vi "oa_Get Angular Speed (N Tach).vi"(7 "reset? (True)":bool=TRUE, 8 "error in (no error)":errorcluster, 9 "durations":dbl[](array[numeric]), 10 "pulse/revolution (1)":i32[](array[numeric]), 11 "pulse position [s]":cluster{dbl[]}[](array[cluster]) {"?" format="%.2f"}) -> (0 "error out":errorcluster, 1 "No Tach? (False)":bool[](array[boolean]), 2 "speed position info":T2[](array[typedef]), 3 "speed profile":T1[](array[typedef]) {"speed [RPM]" format="%.2f"; "time [s]" format="%.2f"})   [LabVIEW 2017, in "SoundVib_TachProcess.lvlib"]
uses:
  <vilib>/addons/Sound and Vibration/Order Analysis/Tach Process/SoundVib_TachProcess.lvlib
  <vilib>/addons/Sound and Vibration/Order Analysis/Misc/OAT Position Info.ctl
  <vilib>/addons/Sound and Vibration/Order Analysis/Tach Process/SubVIs/speed profile.ctl
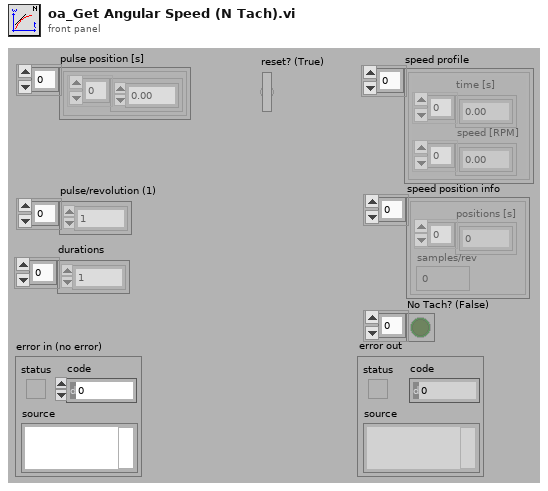
[diagram p1: front panel]
types:
  T1 = typedef "SoundVib_TachProcess.lvlib/speed profile.ctl" = cluster{"time [s]":dbl[], "speed [RPM]":dbl[]}
  T2 = typedef "OAT Position Info.ctl" = cluster{"positions [s]":dbl[], "samples/rev":dbl}
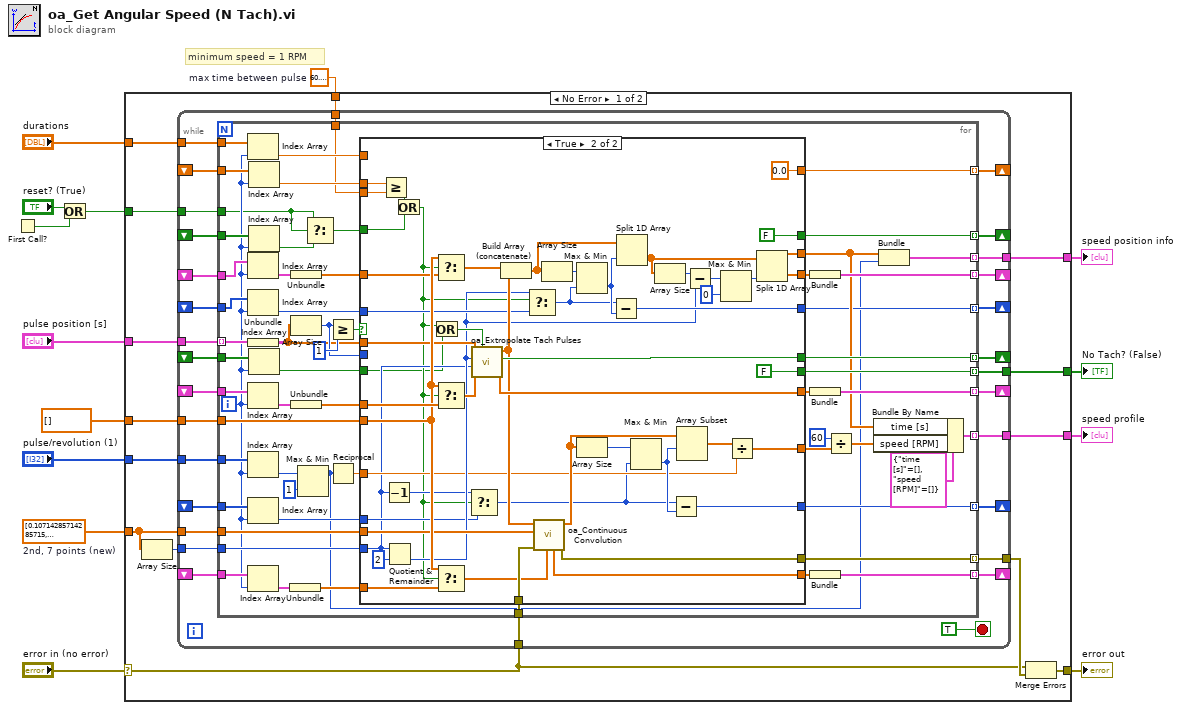
[diagram p0: block diagram]
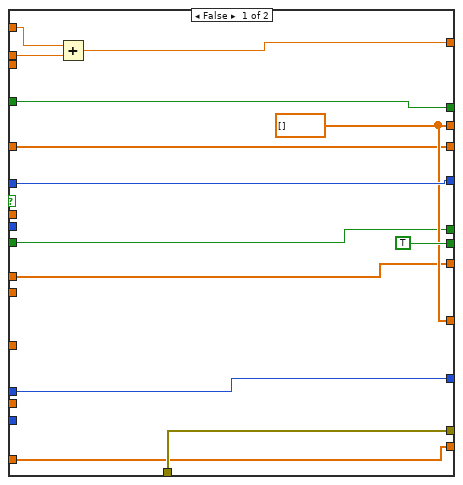
[diagram p2: hidden frame]
diagram:
  w1 = 60.499  # max time between pulse
  w4 = dbl[] [0.10714285714285715, 0.07142857142857142, 0.035714285714285705, -1.5209319782164736e-17, -0.03571428571428571, -0.07142857142857142, -0.10714285714285715]  # 2nd, 7 points (new)
  # "minimum speed = 1 RPM"
  n1 = First Call?() -> (First Call?: T/F=w12:bool)
  n2 = Or(x="reset? (True)", y=w12) -> (x .or. y?=w11:bool)
  n3 = case shown="No Error" "error in (no error)" {
    selector: "error in (no error)" -> [w15 w182]
    tunnel: "pulse position [s]" -> [w28 _]
    tunnel: w11 -> [w27 _]
    tunnel: "pulse/revolution (1)" -> [w26 _]
    tunnel: [w25 _] -> w9
    tunnel: [w24 _] -> w8
    tunnel: [w23 _] -> w7
    tunnel: [w21 w182] -> w6
    tunnel: w4 -> [w20 _]
    tunnel: "durations" -> [w18 _]
    tunnel: dbl[] [] ("t") -> [w17 _]
    tunnel: w1 -> [w16 _]
    frame No Error {
      n4 = Array Size(array=w20) -> (size(s)=w19:i32)
      n5 = while {
        tunnel: w28 -> [w57]
        tunnel: w27 -> [w56]
        tunnel: w26 -> [w55]
        tunnel: [w54] -> w25
        tunnel: [w53] -> w24
        tunnel: [w52] -> w23
        shift-right: [w51] -> _
        shift-left: _ -> [w50]
        shift-right: [w49] -> _
        shift-left: _ -> [w48]
        tunnel: [w47] -> w22
        shift-right: [w46] -> _
        shift-left: _ -> [w45]
        tunnel: w20 -> [w44]
        tunnel: w19 -> [w43]
        shift-right: [w42] -> _
        shift-left: _ -> [w41]
        tunnel: w15 -> [w40]
        shift-right: [w39] -> _
        shift-left: _ -> [w38]
        shift-right: [w37] -> _
        shift-left: _ -> [w36]
        tunnel: w18 -> [w35]
        shift-right: [w34] -> _
        shift-left: _ -> [w33]
        tunnel: w17 -> [w32]
        shift-right: [w30] -> _
        shift-left: _ -> [w31]
        tunnel: w16 -> [w29]
        stop <- TRUE stop-if-true
        n6 = for {
          tunnel: w57 -> [w110] mode=indexing
          tunnel: w56 -> [w65]
          tunnel: w55 -> [w70]
          tunnel: [w108] -> w54 mode=indexing
          tunnel: [w107] -> w53 mode=indexing
          tunnel: [w106] -> w52 mode=indexing
          tunnel: [w100] -> w51 mode=indexing
          tunnel: w50 -> [w105]
          tunnel: [w96] -> w49 mode=indexing
          tunnel: w48 -> [w104]
          tunnel: [w103] -> w47 mode=indexing
          tunnel: [w92] -> w46 mode=indexing
          tunnel: w45 -> [w90]
          tunnel: w44 -> [w88]
          tunnel: w43 -> [w87]
          tunnel: [w86] -> w42 mode=indexing
          tunnel: w41 -> [w72]
          tunnel: w40 -> [w85]
          tunnel: [w83] -> w39 mode=indexing
          tunnel: w38 -> [w82]
          tunnel: [w80] -> w37 mode=indexing
          tunnel: w36 -> [w79]
          tunnel: w35 -> [w77]
          tunnel: [w75] -> w34 mode=indexing
          tunnel: w33 -> [w74]
          tunnel: w32 -> [w68]
          tunnel: w31 -> [w67]
          tunnel: [w62] -> w30 mode=indexing
          tunnel: w29 -> [w60]
          i -> [w66]
          n7 = Index Array(array=w77, index=w66) -> (element=w76:dbl)
          n8 = Index Array(array=w90, index=w66) -> (element=w89:cluster{dbl[]})
          n9 = Index Array(array=w82, index=w66) -> (element=w81:i32)
          n10 = Unbundle(w110) -> (w109:dbl[])
          n11 = Index Array(array=w105, index=w66) -> (element=w99:cluster{"pulse buffer out":dbl[]})
          n12 = Index Array(array=w70, index=w66) -> (element=w69:i32)
          n13 = Index Array(array=w79, index=w66) -> (element=w78:i32)
          n14 = Index Array(array=w104, index=w66) -> (element=w95:cluster{"final state":dbl[]})
          n15 = Index Array(array=w74, index=w66) -> (element=w73:dbl)
          n16 = Index Array(array=w67, index=w66) -> (element=w64:bool)
          n17 = Index Array(array=w72, index=w66) -> (element=w71:bool)
          n18 = Unbundle(w95) -> ("final state"=w94:dbl[])
          n19 = Unbundle(w89) -> (w91:dbl[])
          n20 = Array Size(array=w109) -> (size(s)=w111:i32)
          n21 = Unbundle(w99) -> ("pulse buffer out"=w98:dbl[])
          n22 = Max & Min(x=w69, y=1) -> (max(x,y)=w61:i32)  [unwired: 1 out]
          n23 = Select(t=w65, s=w65, f=w64) -> (s? t:f=w63:bool)
          n24 = Greater Or Equal?(x=w111, y=1) -> (x >= y?=w112:bool)
          n25 = Reciprocal(x=w61) -> (1/x=w117:dbl)
          n26 = case shown="True" w112 {
            tunnel: w117 -> [_ w145]
            tunnel: [w123 w139] -> w114
            tunnel: [w129 w168] -> w103
            tunnel: [TRUE FALSE] -> w106
            tunnel: w111 -> [_ _]
            tunnel: w109 -> [_ w176]
            tunnel: [w121 w173] -> w101
            tunnel: w98 -> [w121 w180]
            tunnel: [w120 w166] -> w97
            tunnel: w94 -> [w120 w179]
            tunnel: [w118 w155] -> w93
            tunnel: w91 -> [w118 w177]
            tunnel: w68 -> [_ w178]
            tunnel: w88 -> [_ w170]
            tunnel: w87 -> [_ w141]
            tunnel: [w119 w172] -> w86
            tunnel: w71 -> [w119 w134]
            tunnel: w85 -> [w129 w169]
            tunnel: [w123 w154] -> w84
            tunnel: [w127 w153] -> w83
            tunnel: w81 -> [w127 w152]
            tunnel: [w128 w144] -> w80
            tunnel: w78 -> [w128 w143]
            tunnel: w76 -> [w126 _]
            tunnel: [w125 0.0] -> w75
            tunnel: w73 -> [w124 w137]
            tunnel: w63 -> [w122 w132]
            tunnel: [w122 FALSE] -> w62
            tunnel: w60 -> [_ w131]
            frame False {
              w123 = dbl[] [] ("pulse history out")
              n27 = Add(x=w126, y=w124) -> (x+y=w125:dbl)
            }
            frame True {
              n28 = Greater Or Equal?(x=w137, y=w131) -> (x >= y?=w136:bool)
              n29 = Decrement(x=w141) -> (x-1=w140:i32)
              n30 = Quotient & Remainder(x=w141, y=2) -> (floor(x/y)=w150:i32)  [unwired: 1 out]
              n31 = Or(x=w136, y=w132) -> (x .or. y?=w135:bool)
              n32 = Or(x=w135, y=w134) -> (x .or. y?=w171:bool)
              n33 = Select(t=w178, s=w135, f=w177) -> (s? t:f=w165:dbl[])
              n34 = Select(t=w178, s=w135, f=w180) -> (s? t:f=w174:dbl[])
              n35 = Select(t=w178, s=w135, f=w179) -> (s? t:f=w167:dbl[])
              n36 = Select(t=w140, s=w135, f=w143) -> (s? t:f=w142:i32)
              n37 = call <vilib>:"oa_Extropolate Tach Pulses.vi"("reset? (True)"=w171, "pulse buffer in"=w174, "modal length"=w141, "extrapolation length"=w150, "pulse in"=w176) -> ("pulse buffer out"=w173:dbl[], "not enough pulses?"=w172:bool, "pulse out"=w164:dbl[])  [unwired: 4 in]
              n38 = Build Array (concatenate)(w165, w164) -> (w156:dbl[])
              n39 = Select(t=w150, s=w135, f=w152) -> (s? t:f=w151:i32)
              n40 = call <vilib>:"oa_Continuous Convolution.vi"("initial state"=w167, "error in (no error)"=w169, "filter coefficients"=w170, "X"=w164) -> ("error out"=w168:errorcluster, "Y"=w146:dbl[], "final state"=w166:dbl[])  [unwired: 5 in]
              n41 = Array Size(array=w156) -> (size(s)=w163:i32)
              n42 = Max & Min(x=w163, y=w151) -> (min(x,y)=w162:i32)  [unwired: 1 out]
              n43 = Array Size(array=w146) -> (size(s)=w149:i32)
              n44 = Subtract(x=w151, y=w162) -> (x-y=w153:i32)
              n45 = Split 1D Array(array=w156, index=w162) -> (second subarray=w161:dbl[])  [unwired: 1 out]
              n46 = Max & Min(x=w149, y=w142) -> (min(x,y)=w147:i32)  [unwired: 1 out]
              n47 = Array Size(array=w161) -> (size(s)=w160:i32)
              n48 = Subtract(x=w142, y=w147) -> (x-y=w144:i32)
              n49 = Array Subset(array=w146, index=w147) -> (w148:dbl[])  [unwired: 1 in]
              n50 = Subtract(x=w160, y=w150) -> (x-y=w159:i32)
              n51 = Max & Min(x=w159, y=0) -> (max(x,y)=w157:i32)  [unwired: 1 out]
              n52 = Divide(x=w148, y=w145) -> (x/y=w139:dbl[])
              n53 = Split 1D Array(array=w161, index=w157) -> (first subarray=w154:dbl[], second subarray=w155:dbl[])
            }
          }
          n54 = Bundle(w93) -> (w92:cluster{dbl[]})  [unwired: 1 in]
          n55 = Bundle("pulse buffer out"=w101) -> (w100:cluster{"pulse buffer out":dbl[]})  [unwired: 1 in]
          n56 = Bundle("final state"=w97) -> (w96:cluster{"final state":dbl[]})  [unwired: 1 in]
          n57 = Divide(x=60, y=w114) -> (x/y=w115:dbl[])
          n58 = Bundle By Name(cluster=T1 {"time [s]"=[], "speed [RPM]"=[]} ("speed profile"), "time [s]"=w84, "speed [RPM]"=w115) -> (w107:T1)
          n59 = Bundle("pulse history out"=w84, w61) -> (w108:cluster{"pulse history out":dbl[], i32})  [unwired: 1 in]
        }
      }
      n60 = Merge Errors(w15, w22) -> (w21:errorcluster)
    }
    frame Error {
    }
  }
  "error out" <- w6
  "speed position info" <- w9
  "No Tach? (False)" <- w7
  "speed profile" <- w8
